vi "Task1.vi"() -> ()   [LabVIEW 2017]
panel:
  out "Leds":bool[](array[boolean])
  in  "Button":bool[](array[boolean])
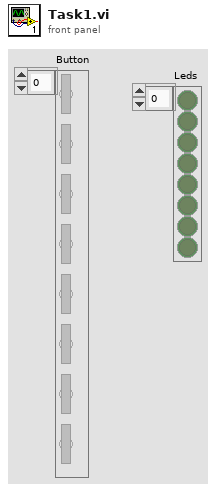
[diagram p1: front panel]
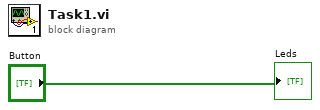
[diagram p0: block diagram]
diagram:
  "Leds" <- "Button"
